vi "Create Control From Variant.vi"(5 "Variant in":variant, 7 "Population":T1=enum."Populate Only", 11 "error in (no error)":errorcluster) -> (4 "Control VI out":refnum<vi>, 8 "Control Reference out":refnum<vi>, 15 "error out":errorcluster)   [LabVIEW 2017, in "Variant Control Scripting.lvlib"]
uses:
  Variant Control Scripting.lvlib
  Control Population Settings.ctl
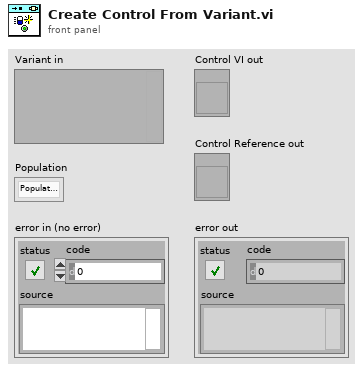
[diagram p1: front panel]
types:
  T1 = typedef "Variant Control Scripting.lvlib/Control Population Settings.ctl" = enum16{"Set Values as Default", "Populate Only", "None"}
  T2 = enum32{"invalid VI type", "Standard VI", "Control VI", "Global VI", "Polymorphic VI", "Configuration VI", "SubSystem", "Facade VI", "Method VI", "Statechart Diagram VI"}
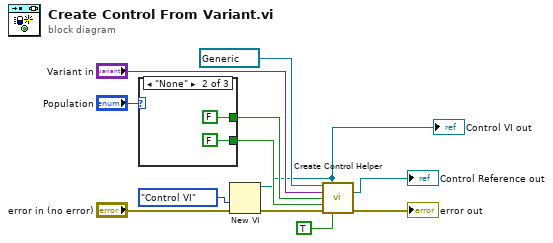
[diagram p0: block diagram]
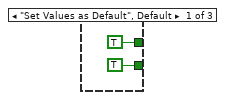
[diagram p2: hidden frame]
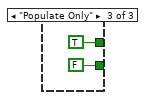
[diagram p3: hidden frame]
diagram:
  n1 = case shown="\"None\"" "Population" {
    tunnel: [TRUE ("add values to arrays") FALSE ("add values to arrays") TRUE ("add values to arrays")] -> w10
    tunnel: [TRUE ("set default values") FALSE ("set default values") FALSE ("set default values")] -> w7
    frame "Set Values as Default", Default {
    }
    frame "None" {
    }
    frame "Populate Only" {
    }
  }
  n2 = New VI(8:"error in (no error)", 9:T2."Control VI" ("vi type (standard vi)")) -> (0:w4:errorcluster, 3:w2:refnum<vi>)  [unwired: 5 in]
  "Control VI out" <- w2
  n3 = call "Create Control Helper.vi"("object refnum"=refnum<vi> refnum, "vi refnum"=w2, "Variant in"="Variant in", "populate values"=w10, "set default values"=w7, "error in (no error)"=w4, "first call?"=TRUE ("use VI refnum")) -> ("Control out"=→"Control Reference out":refnum<vi>, "error out"=→"error out":errorcluster)  [unwired: 7 in]
